vi "Set Parameter Definition.vi"(8 "error in":errorcluster, 10 "parameter definition":T2, 11 "parameter ref in":T1 format="%.0x") -> (0 "error out":errorcluster, 3 "parameter ref out":T1 format="%.0x")   [LabVIEW 2020, in "AIM ARINC 429 Scripting.lvlib"]
uses:
  AIM ARINC 429 Scripting.lvlib
  Shared/Parameter Definition.ctl
  <vilib>/NI/NI VeriStand Encoding and Decoding/Encoding.ctl
  <vilib>/NI VeriStand/Custom Device API/Custom Device Item Ref.ctl
  <vilib>/NI/NI VeriStand Encoding and Decoding/Encoding and Decoding.lvlib
  <vilib>/NI VeriStand/Custom Device API/Custom Device API.lvlib
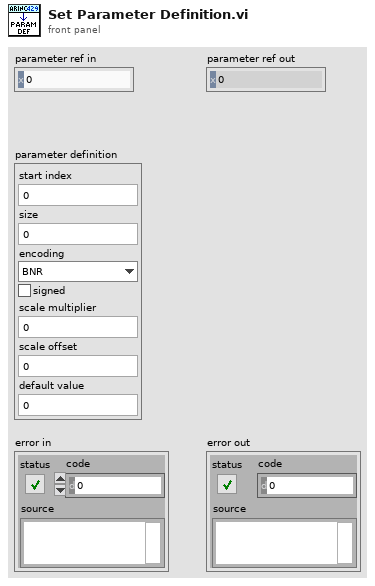
[diagram p1: front panel]
types:
  T1 = typedef "Custom Device API.lvlib/Custom Device Item Ref.ctl" = u64
  T2 = typedef "Parameter Definition.ctl" = cluster{"start index":i32, "size":i32, "encoding":T3, "signed":bool, "scale multiplier":dbl, "scale offset":dbl, "default value":dbl}
  T3 = typedef "Encoding and Decoding.lvlib/Encoding.ctl" = enum16{"BNR", "BCD", "Discrete"}
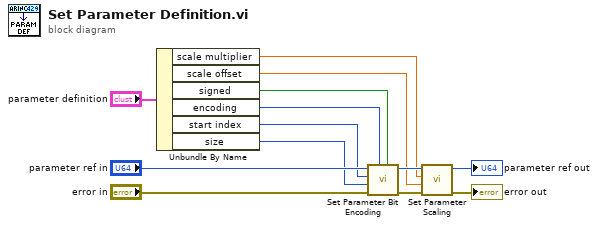
[diagram p0: block diagram]
diagram:
  n1 = Unbundle By Name("parameter definition") -> ("scale multiplier"=w6:dbl, "scale offset"=w5:dbl, "signed"=w4:bool, "encoding"=w3:T3, "start index"=w2:i32, "size"=w1:i32)
  n2 = call "Set Parameter Bit Encoding.vi"("signed?"=w4, "encoding"=w3, "error in"="error in", "number of bits"=w1, "start bit"=w2, "parameter ref in"="parameter ref in") -> ("error out"=w11:errorcluster, "parameter ref out"=w10:T1)  [unwired: 4 in]
  n3 = call "Set Parameter Scaling.vi"("error in"=w11, "scale offset"=w5, "scale multiplier"=w6, "parameter ref in"=w10) -> ("error out"=→"error out":errorcluster, "parameter ref out"=→"parameter ref out":T1)  [unwired: 6 in]
